vi "VI 运行时，当用户在颜色控件上选择了一个颜色后，把前面板上的文字改为相同颜色的文字。.vi"() -> ()   [LabVIEW 2022 SP3]
uses:
  <vilib>/Utility/miscctls.llb/LVTextColorsTypeDef.ctl
panel:
  in  "标题.文本颜色 2":T1 caption="标题.文本颜色"
  in  "标题.文本颜色":T1
  in  "数值 2":dbl caption="重量输入"
  out "变体 2":variant
  in  "输入值的含义 2":enum32{"长度", "重量"}(radio)
  in  "停止 2":bool
  # "英文状态下，ctrl+shift+space 可以呼出快速放置，quick drop"
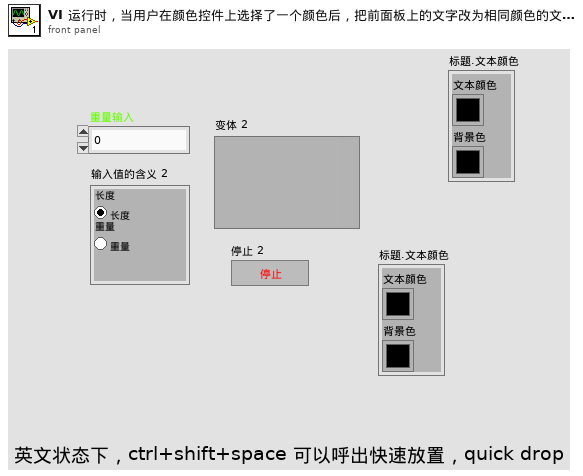
[diagram p1: front panel]
types:
  T1 = typedef "LVTextColorsTypeDef.ctl" = cluster{"Text Color":u32, "Background Color":u32}
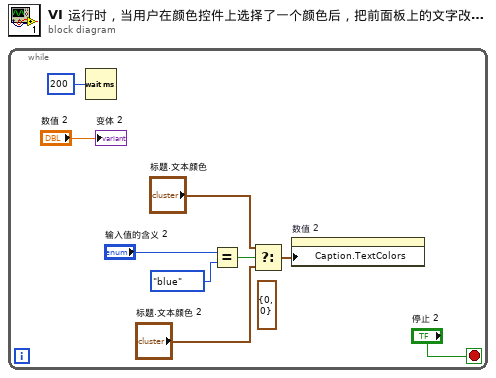
[diagram p0: block diagram]
diagram:
  n1 = while {
    stop <- "停止 2" stop-if-true
    (unwired) T1 {"Text Color"=0, "Background Color"=0} ("标题.文本颜色")
    n2 = Wait (ms)(milliseconds to wait=u32 200 ("等待时间（毫秒）")) -> ()  [unwired: 1 out]
    n3 = Equal?(x="输入值的含义 2", y=enum32{"blue", "red"}."blue") -> (x = y?=w4:bool)
    n4 = Select(t="标题.文本颜色", s=w4, f="标题.文本颜色 2") -> (s? t:f=w1:T1)
    n5 = property on="数值 2" class="DigNum (严格)"("Caption.TextColors"=w1) -> ()  [unwired: 2 in, 2 out]
    "变体 2" <- "数值 2"
  }
